vi "G#Object_VariantToByteArray.vi"(1 "variant":variant) -> (15 "type string":i16[](array[numeric]), 17 "unsigned byte array":u8[](array[numeric]))   [LabVIEW 2017, in "G#Object.lvclass"]
uses:
  G#Object.lvclass
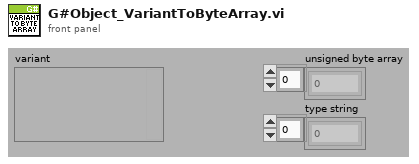
[diagram p1: front panel]
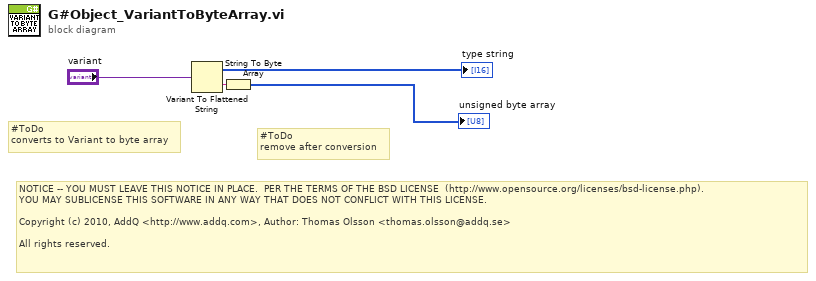
[diagram p0: block diagram]
diagram:
  # "#ToDo\nremove after conversion"
  # "#ToDo\nconverts to Variant to byte array"
  # "NOTICE -- YOU MUST LEAVE THIS NOTICE IN PLACE.  PER THE TERMS OF THE BSD LICENSE  (http://www.opensource.org/licenses/bsd-license.php).\nYOU MAY SUBLICENSE THIS SOFTWARE IN ANY WAY THAT DOES NOT CONFLICT WITH THIS LICENSE.\n\nCopyright (c) 2010, AddQ <http://www.addq.com>, Author: Thomas Olsson <thomas.olsson@addq.se>\n\nAll rights reserved."
  n1 = Variant To Flattened String(Variant="variant") -> (data string=w4:string, 1:→"type string":i16[])
  n2 = String To Byte Array(string=w4) -> (unsigned byte array=→"unsigned byte array":u8[])
